vi "读取数据记录文件.vi"() -> ()   [LabVIEW 2010]
panel:
  in  "选择记录":i32
  out "读取的数据":cluster{string, i32, dbl[]} {"?" format="%.2f"}
  out "读取的采样数据":dbl[](graph)
  # "读取数据记录文件"
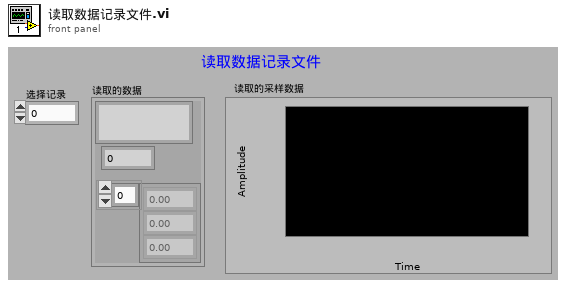
[diagram p1: front panel]
types:
  T1 = cluster{"采样时间":string, "采样率":dbl, "采样数据":dbl[]}[]
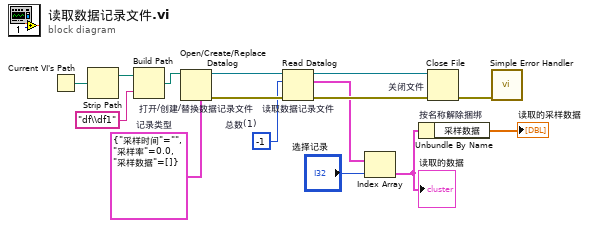
[diagram p0: block diagram]
diagram:
  w4 = -1  # 总数(1)
  w7 = cluster{"采样时间":string, "采样率":dbl, "采样数据":dbl[]} {"采样时间"="", "采样率"=0.0, "采样数据"=[]}  # 记录类型
  n1 = Current VI's Path() -> (path=w10:path)
  n2 = Strip Path(path=w10) -> (stripped path=w9:path)  [unwired: 1 out]
  n3 = Build Path(base path=w9, name or relative path="df\\df1") -> (appended path=w6:path)
  n4 = Open/Create/Replace Datalog "打开/创建/替换数据记录文件"(5:w7, 11:w6) -> (0:w12:errorcluster, 3:w15:refnum<k1>)  [unwired: 4 in, 1 out]
  n5 = Read Datalog "读取数据记录文件"(4:w12, 6:w4, 7:w15) -> (0:w11:errorcluster, 2:w3:T1, 3:w14:refnum<k1>)
  n6 = Index Array(array=w3, index="选择记录") -> (element=w2:cluster{"采样时间":string, "采样率":dbl, "采样数据":dbl[]})
  "读取的数据" <- w2
  n7 = Unbundle By Name "按名称解除捆绑"(w2) -> ("采样数据"=→"读取的采样数据":dbl[])
  n8 = Close File "关闭文件"(refnum=w14, error in=w11) -> (error out=w13:errorcluster)  [unwired: 1 out]
  n9 = call <vilib>:"Simple Error Handler.vi"("error in (no error)"=w13) -> ()  [unwired: 4 in, 5 out]
